vi "read_wav_to_data.vi"(11 "path":path) -> (1 "sampels on file":i32, 2 "UP SAMPLE RATE":fxp<+,48,1>, 3 "wav file out":fxp<+/-,18,1>[](array[numeric]))   [LabVIEW 2021]
panel:
  out "Waveform Graph":waveform(dbl)[](graph)
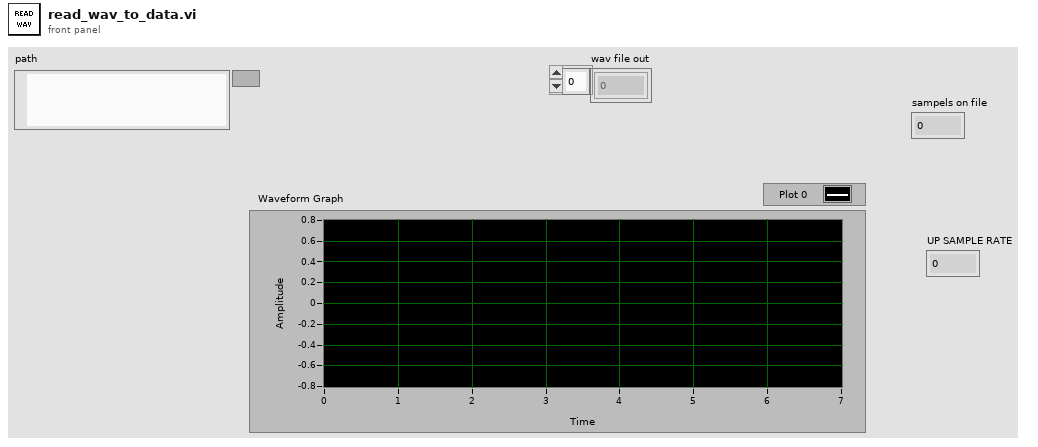
[diagram p1: front panel]
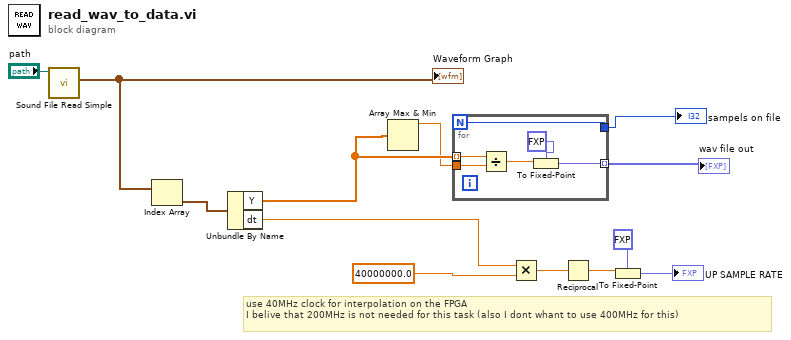
[diagram p0: block diagram]
diagram:
  # "use 40MHz clock for interpolation on the FPGA\nI belive that 200MHz is not needed for this task (also I dont whant to use 400MHz for this)"
  n1 = call <vilib>:"Sound File Read Simple.vi"("path"="path") -> ("data"=w12:waveform(dbl)[])  [unwired: 7 in, 3 out]
  "Waveform Graph" <- w12
  n2 = Index Array(array=w12) -> (element=w11:waveform(dbl))  [unwired: 1 in]
  n3 = Unbundle By Name(w11) -> ("Y"=w8:dbl[], "dt"=w10:dbl)
  n4 = Array Max & Min(array=w8) -> (max value=w7:dbl)  [unwired: 3 out]
  n5 = for {
    N -> [w14]
    tunnel: w8 -> [w19] mode=indexing
    tunnel: w7 -> [w18]
    tunnel: [w15] -> w6 mode=indexing
    tunnel: [w14] -> w5
    n6 = Divide(x=w19, y=w18) -> (x/y=w17:dbl)
    n7 = To Fixed-Point(fixed-point type=fxp<+/-,18,1> 0.0, number=w17) -> (fixed-point=w15:fxp<+/-,18,1>)
  }
  "sampels on file" <- w5
  "wav file out" <- w6
  n8 = Multiply(x=w10, y=40000000.0) -> (x*y=w4:dbl)
  n9 = Reciprocal(x=w4) -> (1/x=w3:dbl)
  n10 = To Fixed-Point(fixed-point type=fxp<+,48,1> 0.0, number=w3) -> (fixed-point=→"UP SAMPLE RATE":fxp<+,48,1>)
